vi "Complex To Cartesian.vi"   [LabVIEW 2020, in "NI_Matrix.lvlib"]
doc: "Breaks a complex number into its rectangular components."
uses:
  <vilib>/Analysis/Matrix/NI_Matrix.lvlib
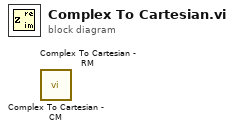
[diagram p0: block diagram]
diagram:
  n1 = call <vilib>:"Complex To Cartesian - CM.vi"() -> ()  [unwired: 1 in, 2 out]
  n2 = call <vilib>:"Complex To Cartesian - RM.vi"() -> ()  [unwired: 1 in, 2 out]
